vi "get information display strings.vi"(8 "error in":errorcluster, 11 "TBM Configuration Node in":refnum<class "TBM Configuration Node.lvclass">) -> (0 "error out":errorcluster, 1 "Data":string[](array[string]), 2 "Labels":string[](array[string]), 3 "TBM Configuration Node out":refnum<class "TBM Configuration Node.lvclass">)   [LabVIEW 2013]
uses:
  TBM Configuration Node.lvclass
  <vilib>/NI/Configuration Framework/serializable configuration/NISE_CEF_serializable configuration.lvclass
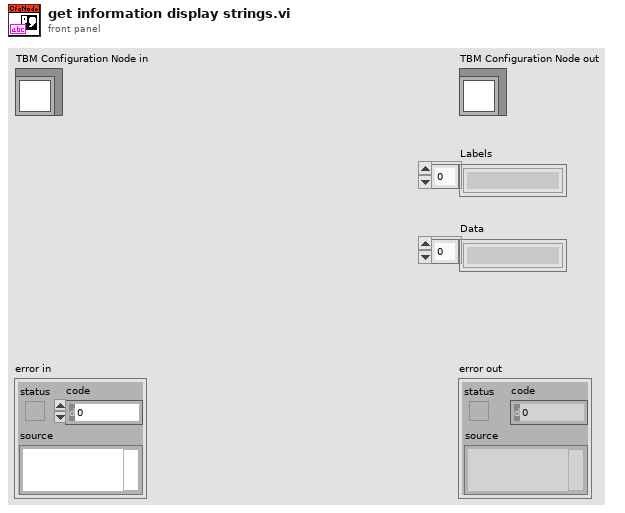
[diagram p1: front panel]
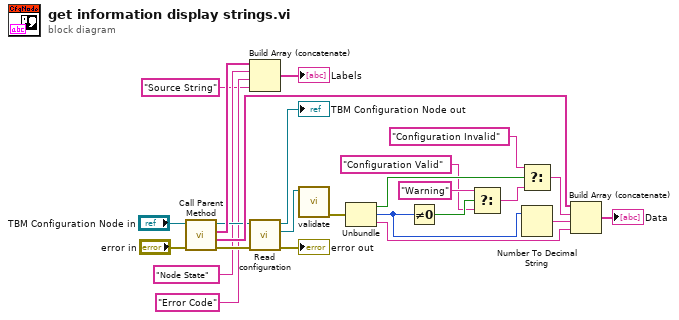
[diagram p0: block diagram]
diagram:
  n1 = call-parent "Call Parent Method"("error in"="error in", "NISE_CEF_serializable node in"="TBM Configuration Node in") -> ("error out"=w25:errorcluster, "Data"=w24:string[], "Labels"=w23:string[], "NISE_CEF_serializable node out"=w18:refnum<class "TBM Configuration Node.lvclass">)  [unwired: 6 in]
  n2 = Build Array (concatenate)(w23, "Node State" ("String"), "Error Code" ("String"), "Source String" ("String")) -> (→"Labels":string[])
  n3 = call-dynamic "Read configuration.vi"("error in"=w25, "NISE_CEF_serializable node in"=w18) -> ("error out"=→"error out":errorcluster, "configuration"=w16:refnum<class "NISE_CEF_serializable configuration.lvclass">, "NISE_CEF_serializable node out"=→"TBM Configuration Node out":refnum<class "TBM Configuration Node.lvclass">)  [unwired: 7 in]
  n4 = call-dynamic "validate.vi"("configuration in"=w16) -> ("error out"=w11:errorcluster)  [unwired: 9 in, 1 out]
  n5 = Unbundle(w11) -> ("status"=w8:bool, "code"=w3:i32, "source"=w1:string)
  n6 = Not Equal To 0?(x=w3) -> (x != 0?=w10:bool)
  n7 = Select(t="Warning" ("String"), s=w10, f="Configuration Valid" ("String")) -> (s? t:f=w7:string)
  n8 = Select(t="Configuration Invalid" ("String"), s=w8, f=w7) -> (s? t:f=w4:string)
  n9 = Number To Decimal String(number=w3) -> (decimal integer string=w2:string)  [unwired: 1 in]
  n10 = Build Array (concatenate)(w24, w4, w2, w1) -> (→"Data":string[])
